vi "Write_Bash.vi"(8 "Time":string, 11 "Test":string="bash wavedump_bash.sh") -> (3 "bash written":bool)   [LabVIEW 2018]
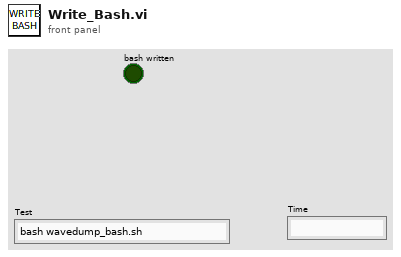
[diagram p1: front panel]
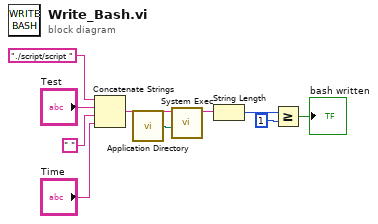
[diagram p0: block diagram]
diagram:
  n1 = Concatenate Strings("./script/script " ("string"), "Test", " " ("string"), "Time") -> (w8:string)
  n2 = call <vilib>:"Application Directory.vi"() -> ("Application Directory"=w5:path)
  n3 = call <vilib>:"System Exec.vi"("working directory"=w5, "command line"=w8) -> ("standard output"=w1:string)  [unwired: 6 in, 3 out]
  n4 = String Length(string=w1) -> (length=w4:i32)
  n5 = Greater Or Equal?(x=w4, y=1) -> (x >= y?=→"bash written":bool)
